vi "MeasurementServer_SetResponse_Config.vi"(0 "gRPCid":T1, 1 "acknowledge":bool, 3 "error in (no error)":errorcluster) -> (10 "error out":errorcluster)   [LabVIEW 2019, in "labview-grpc-measurement-server.lvlib"]
uses:
  labview-grpc-measurement-server.lvlib
  MeasurementServer_gRPCid.ctl
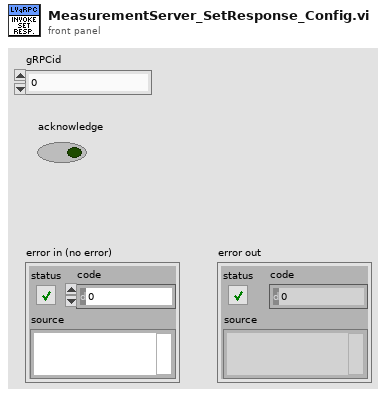
[diagram p1: front panel]
types:
  T1 = typedef "labview-grpc-measurement-server.lvlib/MeasurementServer_gRPCid.ctl" = u64
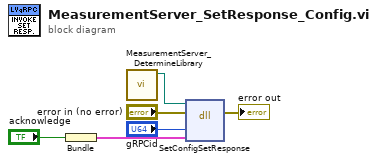
[diagram p0: block diagram]
diagram:
  n1 = Bundle("acknowledge"="acknowledge") -> (w3:cluster{"acknowledge":bool})  [unwired: 1 in]
  n2 = call "MeasurementServer_DetermineLibrary.vi"() -> ("path out"=w1:path)  [unwired: 11 in]
  n3 = dll-call lib="C:/Users/chericks/Desktop/LabVIEW-grpc-measurement-server/build/Debug/labview_measurement_server.dll" fn="SetConfigSetResponse"(path in=w1, error in="error in (no error)", "id"="gRPCid", "data"=w3) -> (error out=→"error out":errorcluster)  [unwired: 4 in, 1 out]
